vi "Refresh Mark Signals To Remove.vi"(8 "error in":errorcluster, 11 "Frame Sysdef":T1 format="%.0x") -> (0 "error out":errorcluster, 3 "Refresh Signals":T2[](array[typedef]))   [LabVIEW 2020, in "Communication Bus Template System Explorer.lvlib" / "Implementation.lvlib"]
uses:
  Types/Refresh Signal.ctl
  <vilib>/NI VeriStand/Custom Device API/Custom Device Item Ref.ctl
  Implementation.lvlib
  Scripting/Communication Bus Template Scripting.lvlib
  <vilib>/NI VeriStand/Custom Device API/Custom Device API.lvlib
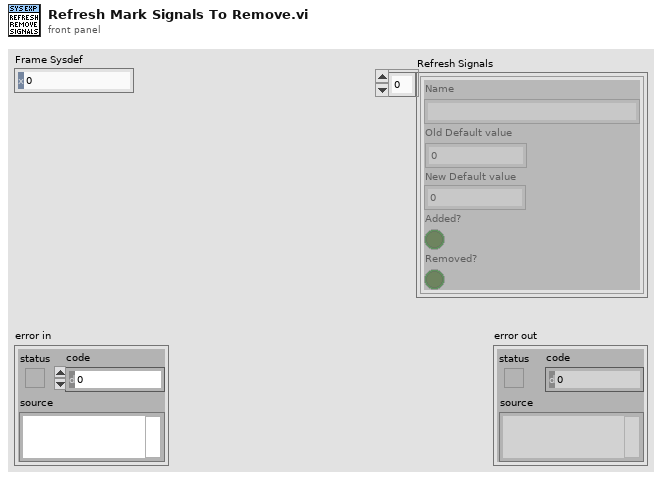
[diagram p1: front panel]
types:
  T1 = typedef "Custom Device API.lvlib/Custom Device Item Ref.ctl" = u64
  T2 = typedef "Communication Bus Template System Explorer.lvlib/Implementation.lvlib/Refresh Signal.ctl" = cluster{"Name":string, "Old Default value":dbl, "New Default value":dbl, "Added?":bool, "Removed?":bool}
  T3 = typedef "Custom Device API.lvlib/Custom Device Channel.ctl" = cluster{"Type":T4, "Units":string, "Default Value":dbl, "Faultable":bool, "Scalable":bool}
  T4 = typedef "Custom Device API.lvlib/Custom Device Channel Type.ctl" = enum16{"Input", "Output"}
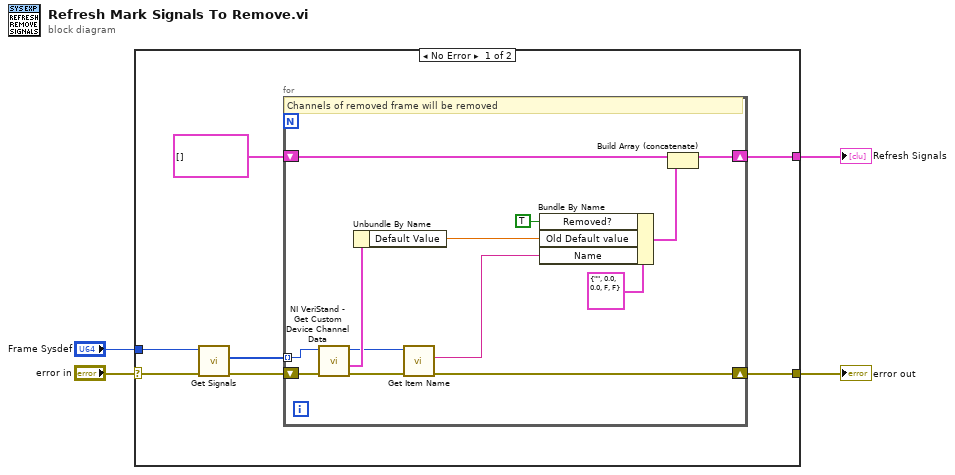
[diagram p0: block diagram]
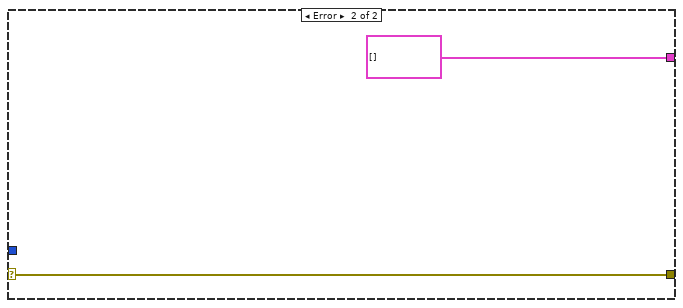
[diagram p2: hidden frame]
diagram:
  n1 = case shown="No Error" "error in" {
    selector: "error in" -> [w7 w26]
    tunnel: [w6 w26] -> w3
    tunnel: [w5 T2[] [] ("Refresh Signals")] -> w2
    tunnel: "Frame Sysdef" -> [w8 _]
    frame No Error {
      n2 = call "Get Signals.vi"("error in"=w7, "Frame in"=w8) -> ("error out"=w11:errorcluster, "Signals"=w10:T1[])  [unwired: 7 in, 1 out]
      n3 = for {
        tunnel: w10 -> [w23] mode=indexing
        shift-right: [w17] -> w6
        shift-left: w11 -> [w24]
        shift-right: [w15] -> w5
        shift-left: T2[] [] ("Refresh Signals") -> [w16]
        # "Channels of removed frame will be removed"
        n4 = call <vilib>:"NI VeriStand - Get Custom Device Channel Data.vi"("error in (no error)"=w24, "Channel Ref in"=w23) -> ("error out"=w20:errorcluster, "Channel"=w22:T3, "Channel Ref out"=w21:T1)  [unwired: 4 in, 3 out]
        n5 = Unbundle By Name(w22) -> ("Default Value"=w18:dbl)
        n6 = call "Get Item Name.vi"("error in"=w20, "Item Ref"=w21) -> ("error out"=w17:errorcluster, "Name"=w19:string)  [unwired: 7 in, 1 out]
        n7 = Bundle By Name(cluster=T2 {"Name"="", "Old Default value"=0.0, "New Default value"=0.0, "Added?"=FALSE, "Removed?"=FALSE} ("Refresh Signal"), "Removed?"=TRUE, "Old Default value"=w18, "Name"=w19) -> (w12:T2)
        n8 = Build Array (concatenate)(w16, w12) -> (w15:T2[])
      }
    }
    frame Error {
    }
  }
  "error out" <- w3
  "Refresh Signals" <- w2
